vi "报警信息插入.vi"(4 "输入字符串":string, 6 "布尔":bool, 7 "Str引用句柄":refnum<vi>) -> (3 "Str引用句柄 2":refnum<vi>)   [LabVIEW 2018]
uses:
  <vilib>/regexp/Match Regular Expression.xnode
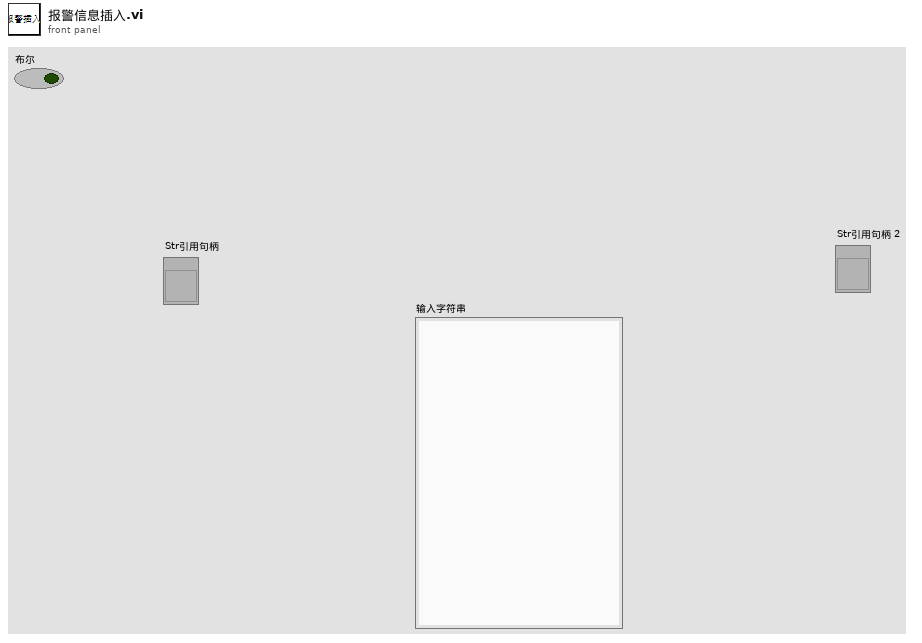
[diagram p1: front panel]
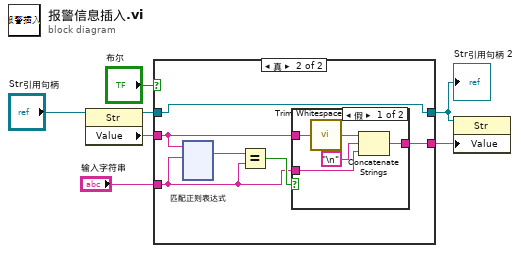
[diagram p0: block diagram]
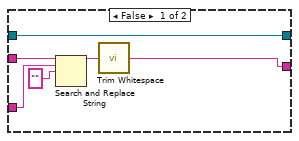
[diagram p2: hidden frame]
diagram:
  n1 = property class="Str"(reference="Str引用句柄") -> (reference out=w2:refnum<vi>, "Value"=w4:string)  [unwired: 1 in, 1 out]
  n2 = case shown="真" "布尔" {
    tunnel: [w9 w17] -> w3
    tunnel: w4 -> [w13 w16]
    tunnel: "输入字符串" -> [w12 w15]
    tunnel: [w8 w14] -> w1
    tunnel: w2 -> [w8 w14]
    frame False {
      n3 = Search and Replace String(input string=w13, search string=w12, replace string="" ("替换字符串(\"\")")) -> (result string=w10:string)  [unwired: 5 in, 3 out]
      n4 = call <vilib>:"Trim Whitespace.vi"("string"=w10) -> ("trimmed string"=w9:string)  [unwired: 1 in]
    }
    frame True {
      n5 = xnode "匹配正则表达式"("输入字符串"=w16, "正则表达式"=w15) -> ("所有匹配"=w19:string)  [unwired: 4 in, 4 out]
      n6 = Equal?(x=w19, y=w15) -> (x = y?=w18:bool)
      n7 = case shown="假" w18 {
        tunnel: [w23 w25] -> w17
        tunnel: w16 -> [w22 w25]
        tunnel: w15 -> [w20 _]
        frame False {
          n8 = call <vilib>:"Trim Whitespace.vi"("string"=w22) -> ("trimmed string"=w21:string)  [unwired: 1 in]
          n9 = Concatenate Strings(w21, "\n", w20) -> (w23:string)
        }
        frame True {
        }
      }
    }
  }
  "Str引用句柄 2" <- w1
  n10 = property class="Str"(reference=w1, "Value"=w3) -> ()  [unwired: 1 in, 2 out]
